vi "configTimingPerChannel.vi"(8 "error in (no error)":errorcluster, 11 "K2602 in":refnum<class "K2602.lvclass">) -> (0 "error out":errorcluster, 3 "K2602 out":refnum<class "K2602.lvclass">)   [LabVIEW 2011, in "Hardware.lvlib" / "Channels.lvlib" / "K2602.lvclass"]
uses:
  K2602.lvclass
  K2602.lvclass/K2602.ctl
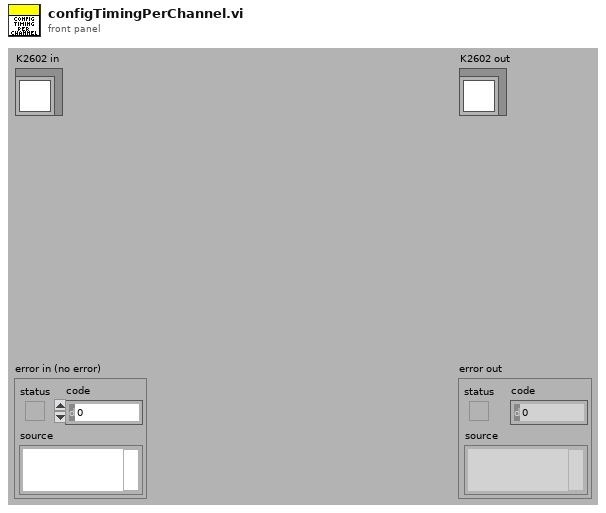
[diagram p1: front panel]
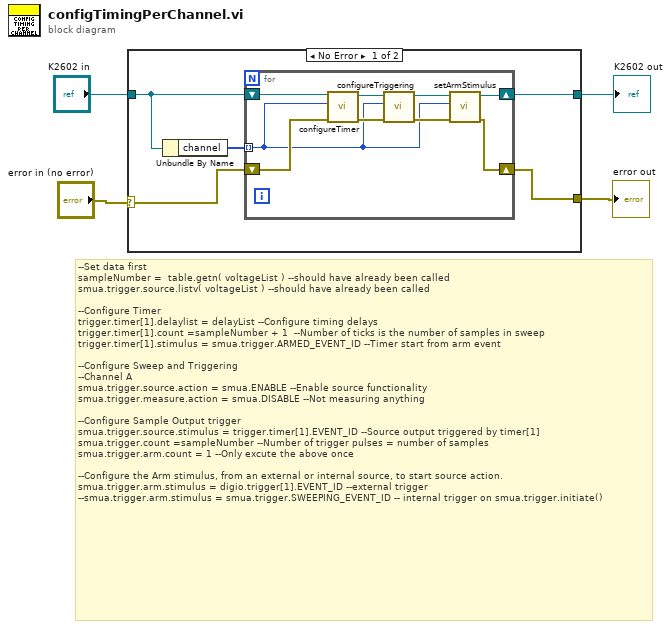
[diagram p0: block diagram]
diagram:
  # "--Set data first\nsampleNumber =  table.getn( voltageList ) --should have already been called\nsmua.trigger.source.listv( voltageList ) --should have already been called\n\n--Configure Timer\ntrigger.timer[1].delaylist = delayList --Configure timing delays\ntrigger.timer[1].count =sampleNumber + 1  --Number of ticks is the number of samples in sweep\ntrigger.timer[1].stimulus = smua.trigger.ARMED_EVENT_ID --Timer start from arm event\n\n--Configure Sweep and Triggering\n--Channel A\nsmua.trigger.source.action = smua.ENABLE --Enable source functionality\nsmua.trigger.measure.action = smua.DISABLE --Not measuring anything\n\n--Configure Sample Output trigger\nsmua.trigger.source.stimulus = trigger.timer[1].EVENT_ID --Source output triggered by timer[1]\nsmua.trigger.count =sampleNumber --Number of trigger pulses = number of samples\nsmua.trigger.arm.count = 1 --Only excute the above once\n\n--Configure the Arm stimulus, from an external or internal source, to start source action.\nsmua.trigger.arm.stimulus = digio.trigger[1].EVENT_ID --external trigger\n--smua.trigger.arm.stimulus = smua.trigger.SWEEPING_EVENT_ID -- internal trigger on smua.trigger.initiate()"
  n1 = case shown="No Error" "error in (no error)" {
    selector: "error in (no error)" -> [w7 w19]
    tunnel: "K2602 in" -> [w8 w20]
    tunnel: [w6 w20] -> w2
    tunnel: [w5 w19] -> w1
    frame No Error {
      n2 = Unbundle By Name(w8) -> ("channel"=w9:i32[])
      n3 = for {
        tunnel: w9 -> [w10] mode=indexing
        shift-right: [w12] -> w6
        shift-left: w8 -> [w18]
        shift-right: [w11] -> w5
        shift-left: w7 -> [w17]
        n4 = call "configureTimer.vi"("error in (no error)"=w17, "channel"=w10, "K2602 in"=w18) -> ("error out"=w15:errorcluster, "K2602 out"=w16:refnum<class "K2602.lvclass">)  [unwired: 7 in]
        n5 = call "configureTriggering.vi"("error in (no error)"=w15, "channel"=w10, "K2602 in"=w16) -> ("error out"=w13:errorcluster, "K2602 out"=w14:refnum<class "K2602.lvclass">)  [unwired: 7 in]
        n6 = call "setArmStimulus.vi"("error in (no error)"=w13, "channel"=w10, "K2602 in"=w14) -> ("error out"=w11:errorcluster, "K2602 out"=w12:refnum<class "K2602.lvclass">)  [unwired: 7 in]
      }
    }
    frame Error {
    }
  }
  "error out" <- w1
  "K2602 out" <- w2
